vi "EMA IIR.vi"(0 "input":fxp<+/-,48,1>, 1 "reset":bool, 5 "b_n":i8, 9 "input valid":bool) -> (4 "output":fxp<+/-,48,1>, 10 "output valid":bool)   [LabVIEW 2017, in "NI PLL IP FPGA.lvlib"]
uses:
  NI PLL IP FPGA.lvlib
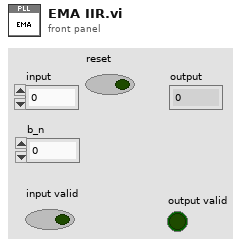
[diagram p1: front panel]
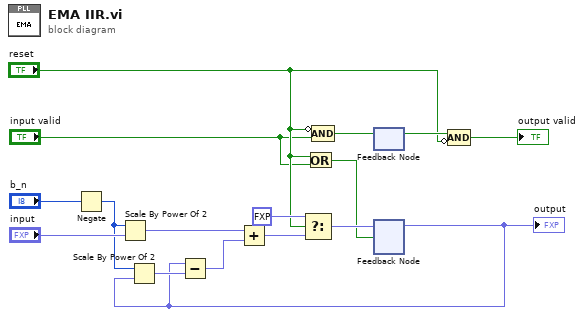
[diagram p0: block diagram]
diagram:
  n1 = Negate(x="b_n") -> (-x=w13:i8)
  n2 = Scale By Power Of 2(n=w13, x="input") -> (x*2^n=w14:fxp<+/-,48,1>)
  n3 = Or(x="reset", y="input valid") -> (x .or. y?=w1:bool)
  n4 = Compound Arithmetic op=AND(invert "reset", "input valid") -> (w8:bool)
  n5 = feedback-in #1(w8) -> ()
  n6 = feedback #1() -> (w7:bool)  [unwired: 1 in]
  n7 = feedback #2() -> (w9:fxp<+/-,48,1>)  [unwired: 1 in]
  "output" <- w9
  n8 = Scale By Power Of 2(n=w13, x=w9) -> (x*2^n=w12:fxp<+/-,48,1>)
  n9 = Subtract(x=w9, y=w12) -> (x-y=w11:fxp<+/-,49,2>)
  n10 = Add(x=w14, y=w11) -> (x+y=w10:fxp<+/-,48,1>)
  n11 = Select(t=fxp<+/-,48,1> 0.0, s="reset", f=w10) -> (s? t:f=w5:fxp<+/-,48,1>)
  n12 = feedback-in #2(w5, w1) -> ()
  n13 = Compound Arithmetic op=AND(w7, invert "reset") -> (→"output valid":bool)
